vi "Init GUI Objects.vi"(8 "Error In":errorcluster, 11 "GUI Object References":T1) -> (0 "Error Out":errorcluster)   [LabVIEW 2016, in "Error Manager.lvlib"]
doc: "This VI configures the \"look and feel\" of GUI objects, and sets their initial value (their contents)."
uses:
  Error Manager.lvlib
  Display Order Combo Box/Display Order Combo Box.lvclass
  Multi-Column Listbox/MCL.lvclass
  Mark Selected Errors As Read Button/Mark Selected Errors As Read Button.lvclass
  Mark All Errors As Read Button/Mark All Errors As Read Button.lvclass
  Settings/Settings.lvclass
  GUI Object References (cluster).ctl
panel:
  out "Initial MCL Value":i32[](array[numeric])
  # "Development\nControls or indicators that are useful for development or testing, but which are not outputs of the VI."
  # "Input\nInputs to the VI"
  # "Output\nOutputs of the VI"
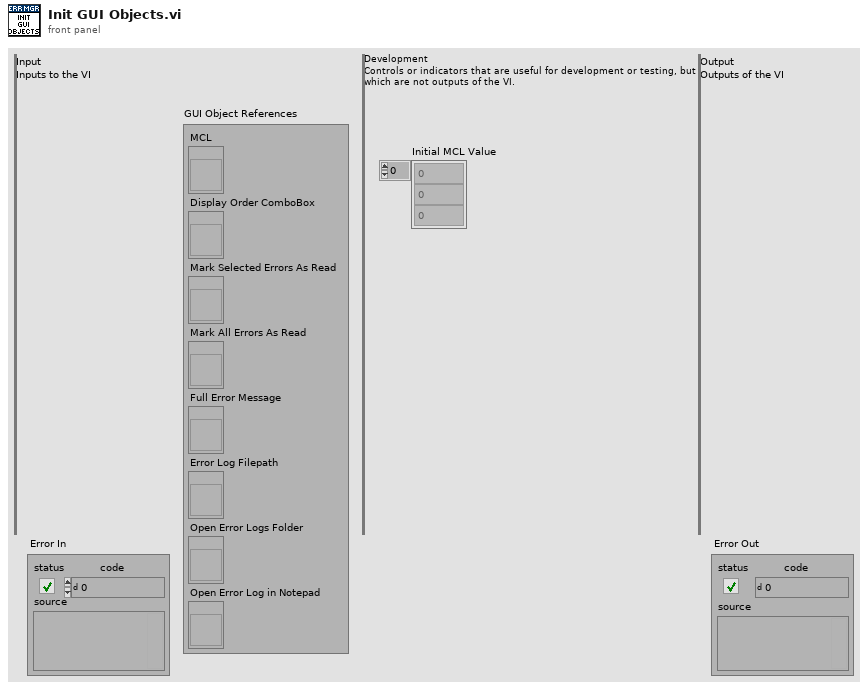
[diagram p1: front panel]
types:
  T1 = typedef "Error Manager.lvlib/GUI Object References (cluster).ctl" = cluster{"MCL":refnum<vi>, "Display Order ComboBox":refnum<vi>, "Mark Selected Errors As Read":refnum<vi>, "Mark All Errors As Read":refnum<vi>, "Full Error Message":refnum<vi>, "Error Log Filepath":refnum<vi>, "Open Error Logs Folder":refnum<vi>, "Open Error Log in Notepad":refnum<vi>}
  T2 = typedef "Error Manager.lvlib/Settings.lvclass/Error_Log_Setting (enum).ctl" = enum16{"Log Full Error Details", "Log Error Codes Only", "Do Not Log"}
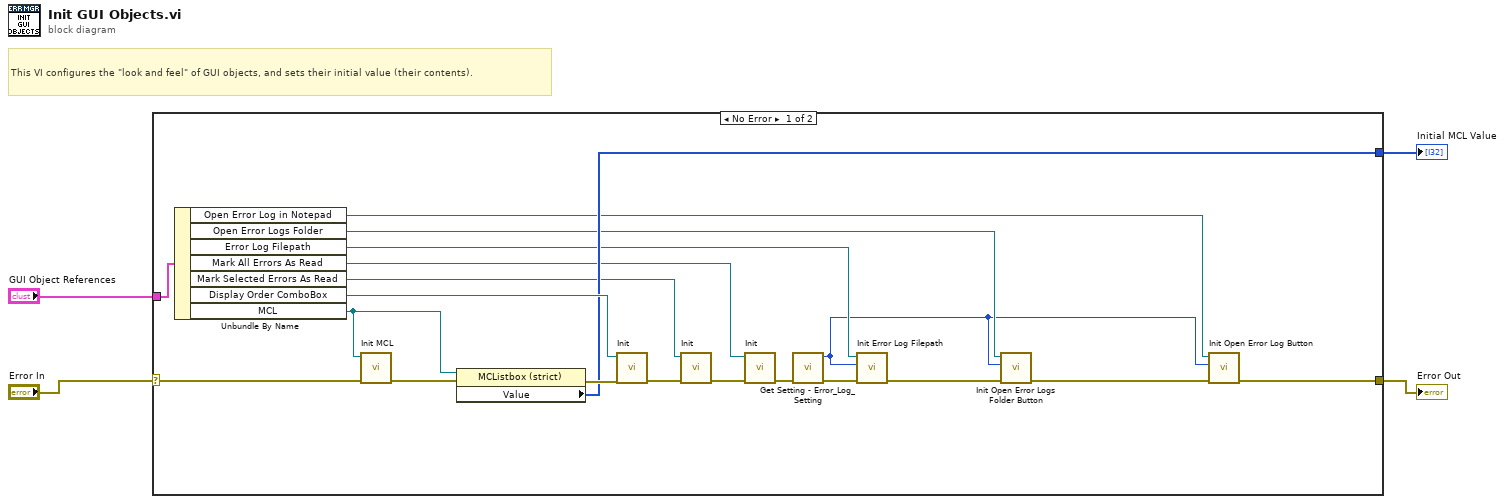
[diagram p0: block diagram]
diagram:
  # "This VI configures the \"look and feel\" of GUI objects, and sets their initial value (their contents)."
  n1 = case shown="No Error" "Error In" {
    selector: "Error In" -> [w24 w25]
    tunnel: [w7 w25] -> w3
    tunnel: "GUI Object References" -> [w23 _]
    tunnel: [w17 _] -> w1
    frame No Error {
      n2 = Unbundle By Name(w23) -> ("Open Error Log in Notepad"=w6:refnum<vi>, "Open Error Logs Folder"=w9:refnum<vi>, "Error Log Filepath"=w12:refnum<vi>, "Mark All Errors As Read"=w14:refnum<vi>, "Mark Selected Errors As Read"=w15:refnum<vi>, "Display Order ComboBox"=w22:refnum<vi>, "MCL"=w20:refnum<vi>)
      n3 = call "Init MCL.vi"("error in (no error)"=w24, "MCL Reference"=w20) -> ("error out"=w21:errorcluster)  [unwired: 9 in]
      n4 = property class="MCListbox (strict)"(reference=w20, error in=w21) -> (error out=w18:errorcluster, "Value"=w17:i32[])  [unwired: 1 out]
      n5 = call "Init.vi"("error in (no error)"=w18, "ComboBox Ref"=w22) -> ("error out"=w16:errorcluster)  [unwired: 9 in]
      n6 = call "Init.vi"("error in (no error)"=w16, "Mark Selected Errors As Read Button Reference"=w15) -> ("error out"=w19:errorcluster)  [unwired: 9 in]
      n7 = call "Init.vi"("error in (no error)"=w19, "Mark All Errors As Read Button Reference"=w14) -> ("error out"=w13:errorcluster)  [unwired: 9 in]
      n8 = call "Get Setting - Error_Log_Setting.vi"("Error In"=w13) -> ("Error Out"=w11:errorcluster, "Error_Log_Setting"=w5:T2)  [unwired: 9 in]
      n9 = call "Init Error Log Filepath.vi"("error in (no error)"=w11, "Error_Log_Setting"=w5, "Error Log Filepath Reference"=w12) -> ("error out"=w10:errorcluster)  [unwired: 8 in]
      n10 = call "Init Open Error Logs Folder Button.vi"("error in (no error)"=w10, "Error_Log_Setting"=w5, "Open Error Logs Folder Button Reference"=w9) -> ("error out"=w8:errorcluster)  [unwired: 8 in]
      n11 = call "Init Open Error Log Button.vi"("error in (no error)"=w8, "Error_Log_Setting"=w5, "\"Open Error Log in Notepad\" Button Reference"=w6) -> ("error out"=w7:errorcluster)  [unwired: 8 in]
    }
    frame Error {
    }
  }
  "Error Out" <- w3
  "Initial MCL Value" <- w1
